vi "Identify.vi"(8 "error in (no error)":errorcluster, 11 "Square in":refnum<class "Square.lvclass">) -> (0 "error out":errorcluster, 2 "Class name":string, 3 "Square out":refnum<class "Square.lvclass">)   [LabVIEW 2023, in "Square.lvclass"]
doc: "This VI is a method that demonstrates dynamic dispatching."
uses:
  Square.lvclass
panel:
  in  "Class name (constant)":string="Square"
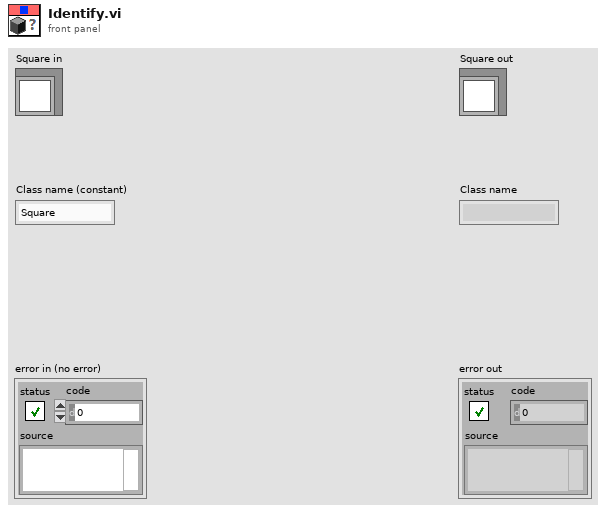
[diagram p1: front panel]
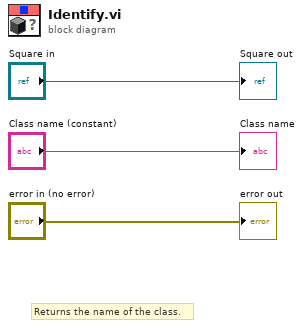
[diagram p0: block diagram]
diagram:
  # "Returns the name of the class."
  "error out" <- "error in (no error)"
  "Square out" <- "Square in"
  "Class name" <- "Class name (constant)"
